vi "Get Build Specifications.vi"(8 "error in (no error)":errorcluster, 11 "Project Path in":path) -> (0 "error out":errorcluster, 2 "Build Specification Names":string[](array[string]), 3 "Project Path out":path)   [LabVIEW 2019, in "Package Builder.lvlib"]
uses:
  Package Builder.lvlib
panel:
  in  "Project Path":path
  in  "Build Specification Name":string
  in  "Target Name":string
  in  "Top Level/Always Included VIs":path[](array[path])
  in  "Main Destination Path":path
  out "Build Specification Names":string[](array[string])
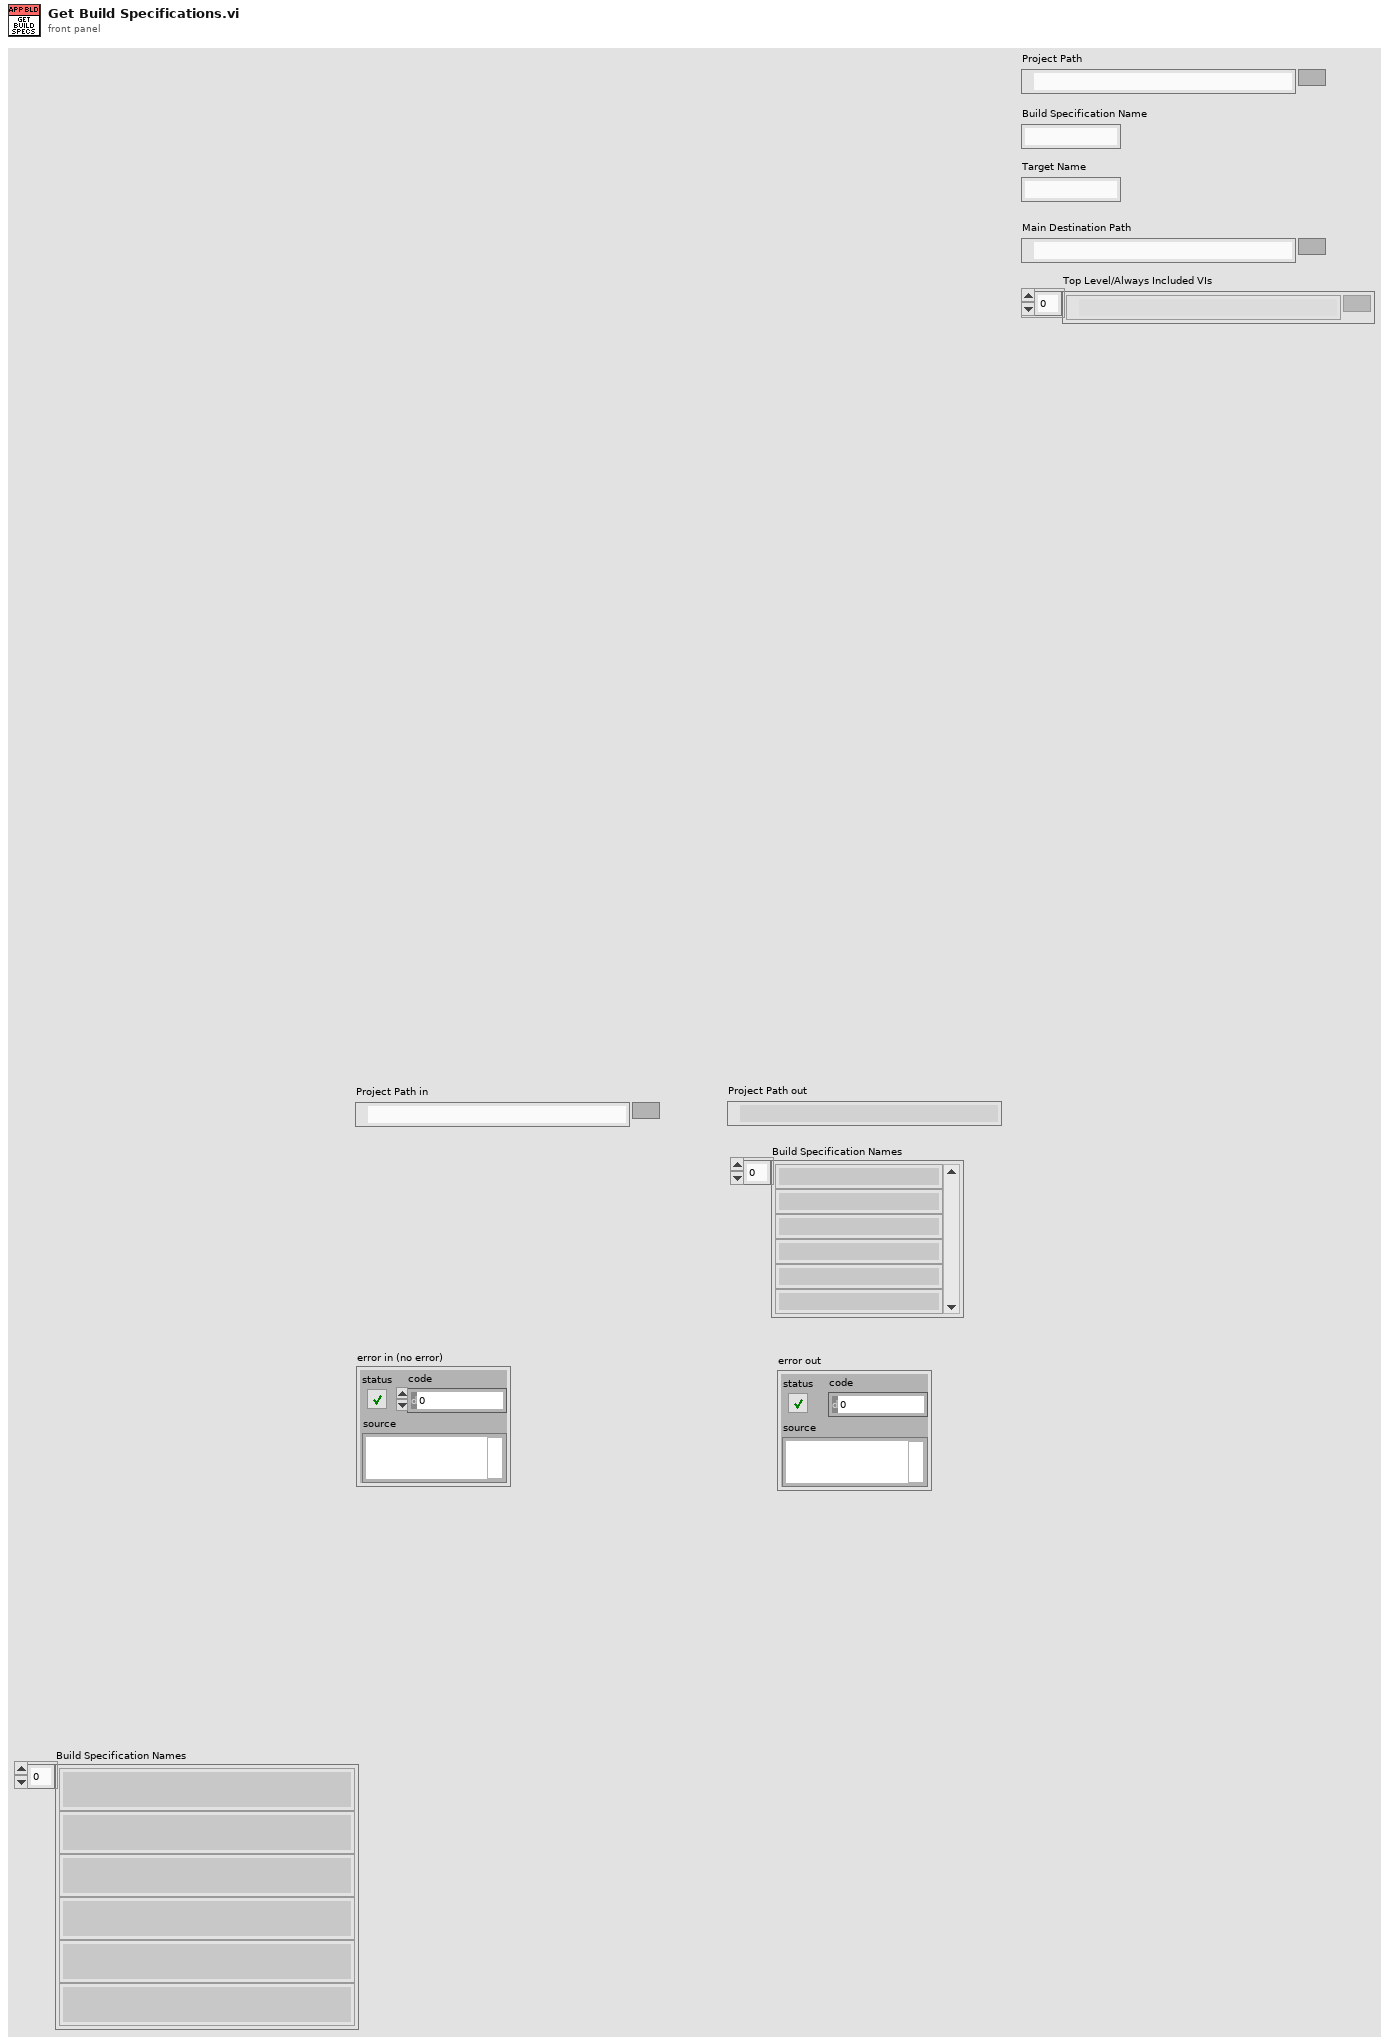
[diagram p1: front panel]
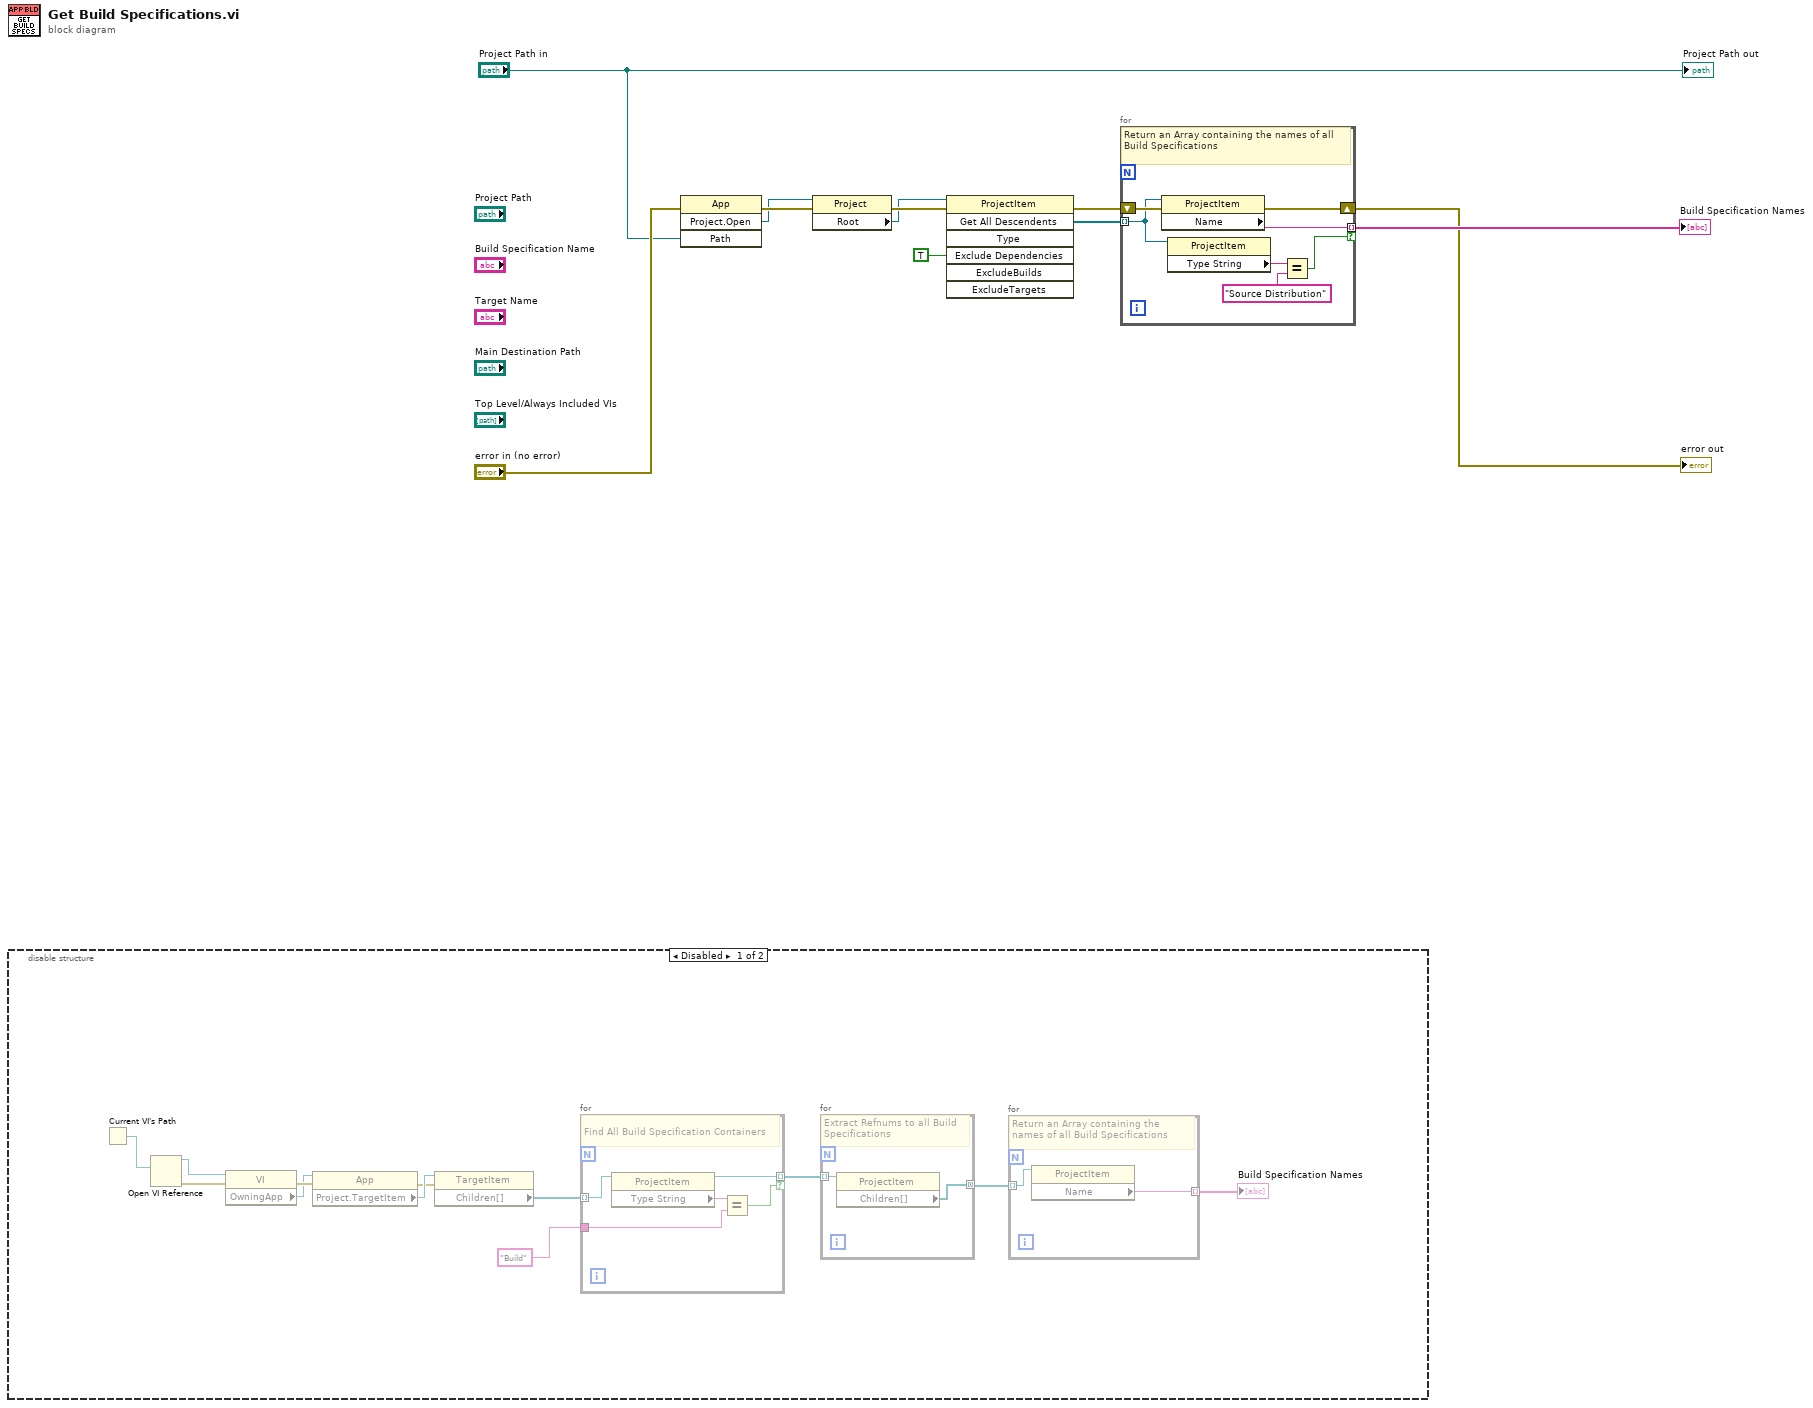
[diagram p0: block diagram]
diagram:
  n1 = disable-structure shown="Disabled" {
    frame Disabled {
      n2 = Current VI's Path() -> (path=w14:path)
      n3 = Open VI Reference(vi path=w14) -> (vi reference=w15:refnum<vi>, error out=w16:errorcluster)  [unwired: 5 in]
      n4 = property class="VI"(reference=w15, error in=w16) -> (error out=w22:errorcluster, "OwningApp"=w17:refnum<vi>)  [unwired: 1 out]
      n5 = property class="App"(reference=w17, error in=w22) -> (error out=w18:errorcluster, "Project.TargetItem"=w19:refnum<vi>)  [unwired: 1 out]
      n6 = property class="TargetItem"(reference=w19, error in=w18) -> ("Children[]"=w20:refnum<vi>[])  [unwired: 2 out]
      n7 = for {
        tunnel: w20 -> [w32] mode=indexing
        tunnel: [w30] -> w21 mode=indexing if=w29
        tunnel: "Build" ("y") -> [w28]
        # "Find All Build Specification Containers"
        n8 = property class="ProjectItem"(reference=w32) -> (reference out=w30:refnum<vi>, "Type String"=w31:string)  [unwired: 1 in, 1 out]
        n9 = Equal?(x=w31, y=w28) -> (x = y?=w29:bool)
      }
      n10 = for {
        tunnel: w21 -> [w27] mode=indexing
        tunnel: [w26] -> w12 mode=concatenating
        # "Extract Refnums to all Build Specifications"
        n11 = property class="ProjectItem"(reference=w27) -> ("Children[]"=w26:refnum<vi>[])  [unwired: 1 in, 2 out]
      }
      n12 = for {
        tunnel: w12 -> [w25] mode=indexing
        tunnel: [w24] -> w13 mode=indexing
        # "Return an Array containing the names of all Build Specifications"
        n13 = property class="ProjectItem"(reference=w25) -> ("Name"=w24:string)  [unwired: 1 in, 2 out]
      }
      "Build Specification Names" <- w13
    }
    frame Enabled {
    }
  }
  n14 = invoke class="App" method="Project.Open"(error in="error in (no error)", "Path"="Project Path in") -> (error out=w8:errorcluster, "Project:Open"=w7:refnum<vi>)  [unwired: 2 in, 2 out]
  n15 = property class="Project"(reference=w7, error in=w8) -> (error out=w10:errorcluster, "Root"=w9:refnum<vi>)  [unwired: 1 out]
  n16 = invoke class="ProjectItem" method="Get All Descendents"(reference=w9, error in=w10, "Exclude Dependencies"=TRUE ("ExcludeDependencies")) -> (error out=w5:errorcluster, "All Descendents"=w6:refnum<vi>[])  [unwired: 4 in, 5 out]
  n17 = for {
    tunnel: w6 -> [w36] mode=indexing
    tunnel: [w39] -> w4 mode=indexing if=w33
    shift-right: [w37] -> w2
    shift-left: w5 -> [w38]
    # "Return an Array containing the names of all Build Specifications"
    n18 = property class="ProjectItem"(reference=w36, error in=w38) -> (error out=w37:errorcluster, "Name"=w39:string)  [unwired: 1 out]
    n19 = property class="ProjectItem"(reference=w36) -> ("Type String"=w35:string)  [unwired: 1 in, 2 out]
    n20 = Equal?(x=w35, y="Source Distribution") -> (x = y?=w33:bool)
  }
  "Build Specification Names" <- w4
  "error out" <- w2
  "Project Path out" <- "Project Path in"
